vi "Actor Core.vi"(8 "error in":errorcluster, 11 "Apply Language Wizard in":refnum<class "Apply Language Wizard.lvclass">) -> (0 "error out":errorcluster, 3 "Actor out":refnum<class "Actor.lvclass">)   [LabVIEW 2013, in "SET Project Editor.lvlib" / "Apply Language Wizard.lvclass"]
doc: "(<B>Filename</B>: Actor Framework.lvlib:Actor.lvclass:Actor Core.vi)\n\nReceives messages to the actor, reacts to them, and initiates any error handling that may shut the actor down.\n\nDescendant classes may override this VI to append parallel tasks for the actor to complete while it handles messages. Overrides use the Call Parent Method node."
uses:
  Apply Language Wizard.lvclass
  <vilib>/ActorFramework/Actor/Actor.lvclass
  <vilib>/ActorFramework/Actor/Actor.lvclass/Actor.ctl
  <vilib>/ActorFramework/Message Enqueuer/Message Enqueuer.lvclass/Message Enqueuer.ctl
  Apply Language Wizard.lvclass/Apply Language Wizard.ctl
  lib/printf/messages/General/LV_Printf Msg.lvclass/LV_Printf Msg.ctl
  UI Wizard/UI Wizard.lvclass
  lib/printf/messages/General/Read Message.vi
  <vilib>/ActorFramework/Message Enqueuer/Init from Existing Queue.vi
  <vilib>/ActorFramework/Message Enqueuer/Enqueue.vi
  <vilib>/ActorFramework/Message Priority Queue/Priority Enqueue.vi
  <vilib>/ActorFramework/Message Enqueuer/Message Enqueuer.lvclass
  <vilib>/ActorFramework/Stop Msg/Stop Msg.lvclass
  Apply Language Wizard Messages/Apply Language to Project Msg/Apply Language to Project Msg.lvclass
  lib/printf/Core/LV_Printf Core.lvclass
  lib/printf/messages/General/LV_Printf Msg.lvclass
panel:
  in  "Tab Control":enum32{"Page 1", "Page 2"}(tab)
  in  "Next1":bool
  out "Project Name":string
  in  "Cancel1":bool
  in  "Target Language":string(combo)="en" caption="Default Language"
  in  "VI Selector":i32(listbox)
  in  "RTM Selector":i32(listbox)
  out "Status":string
  in  "Finish":bool
  in  "Cancel2":bool
  # "Apply Language Wizard"
  # "Select VIs"
  # "Select Run-Time Menus"
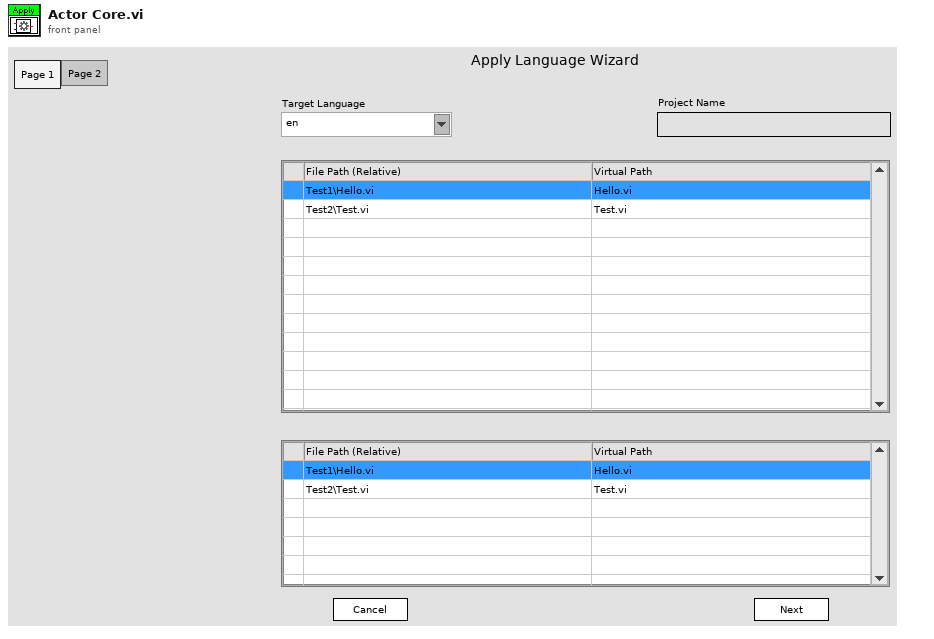
[diagram p1: front panel]
types:
  T1 = typedef "LVPoint32TypeDef.ctl" = cluster{"Horizontal":i32, "Vertical":i32}
  T2 = typedef "LVRowAndColumnTypeDef.ctl" = cluster{"Row":i32, "Column":i32}
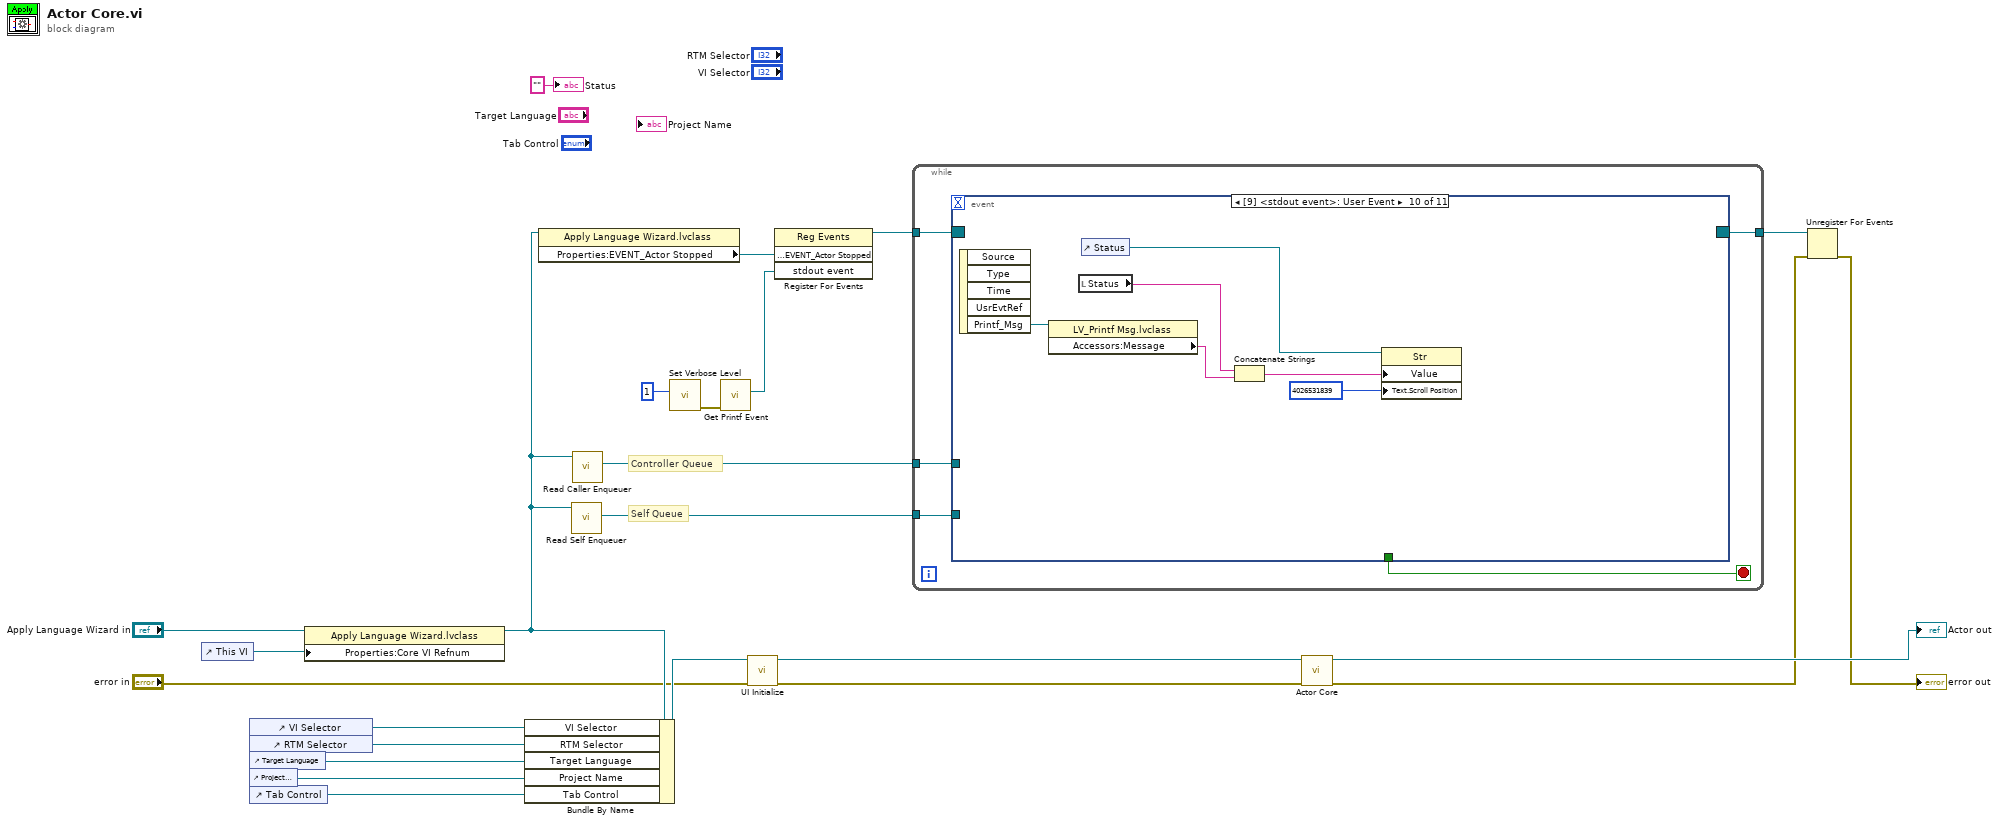
[diagram p0: block diagram]
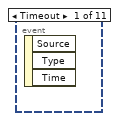
[diagram p2: hidden frame]
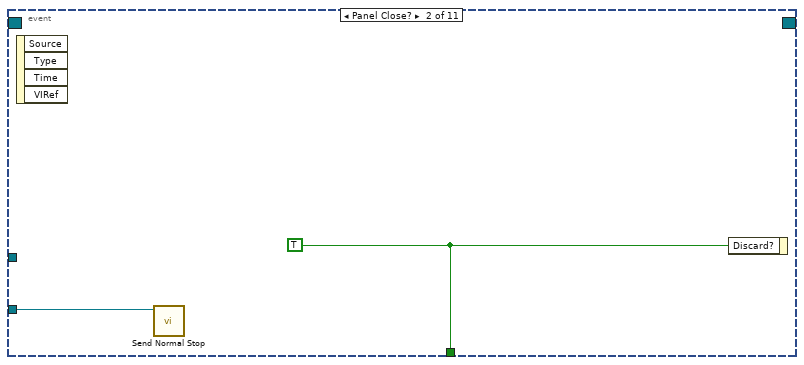
[diagram p3: hidden frame]
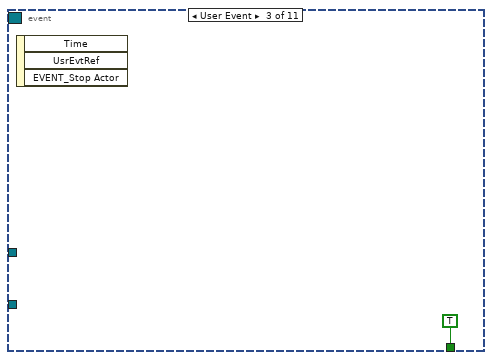
[diagram p4: hidden frame]
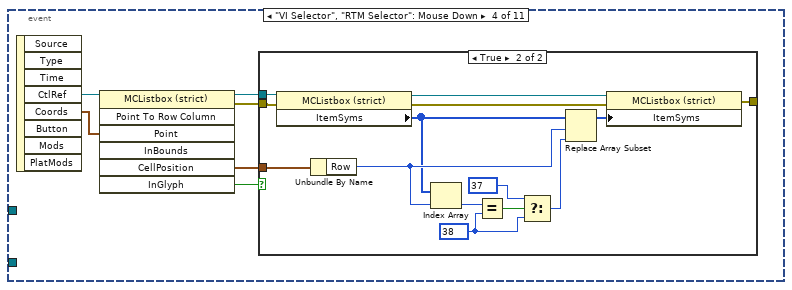
[diagram p5: hidden frame]
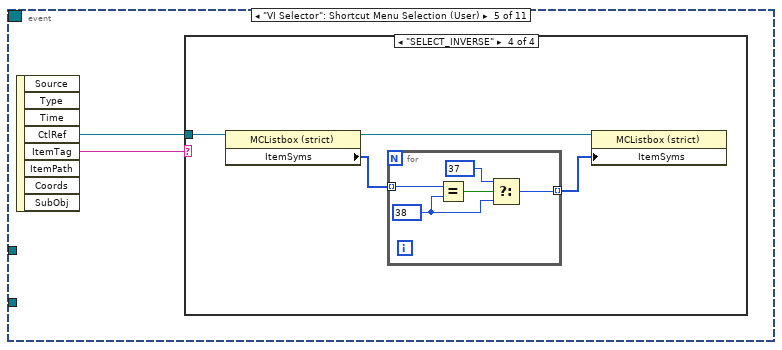
[diagram p7: hidden frame]
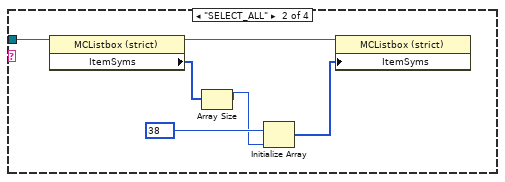
[diagram p9: hidden frame]
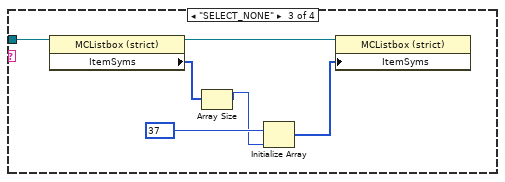
[diagram p10: hidden frame]
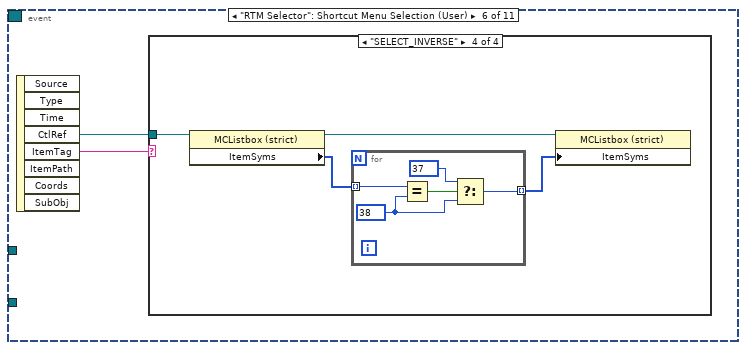
[diagram p11: hidden frame]
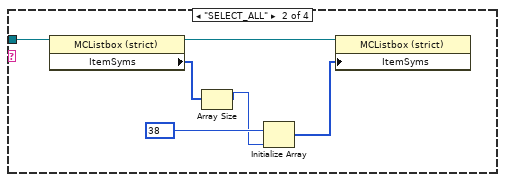
[diagram p13: hidden frame]
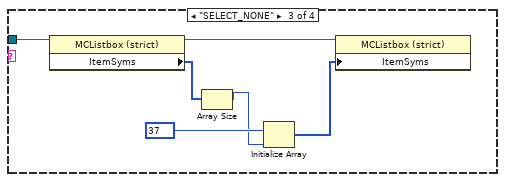
[diagram p14: hidden frame]
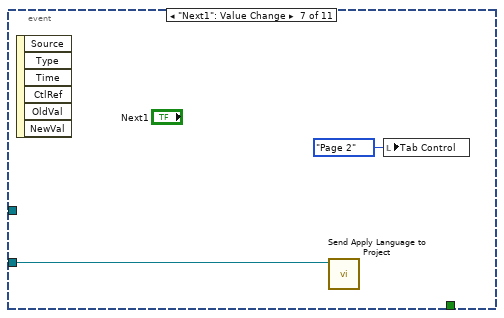
[diagram p15: hidden frame]
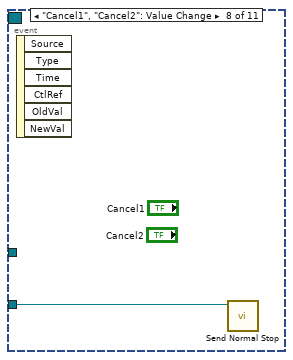
[diagram p16: hidden frame]
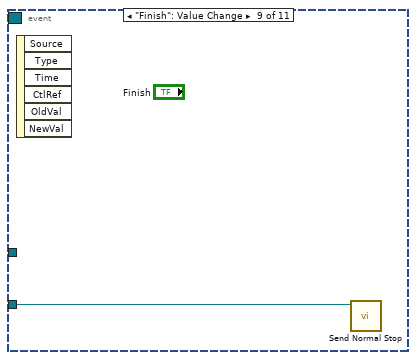
[diagram p17: hidden frame]
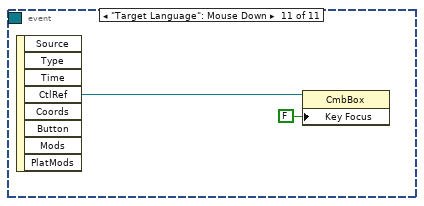
[diagram p18: hidden frame]
diagram:
  # "Controller Queue"
  # "Self Queue"
  n1 = control-ref of="This VI"() -> (w18:refnum<vi>)
  n2 = control-ref of="VI Selector"() -> (w3:refnum<vi>)
  n3 = control-ref of="RTM Selector"() -> (w4:refnum<vi>)
  n4 = control-ref of="Target Language"() -> (w5:refnum<vi>)
  n5 = control-ref of="Project Name"() -> (w2:refnum<vi>)
  n6 = control-ref of="Tab Control"() -> (w6:refnum<vi>)
  n7 = property class="Apply Language Wizard.lvclass"(reference="Apply Language Wizard in", "Properties:Core VI Refnum"=w18) -> (reference out=w9:refnum<class "Apply Language Wizard.lvclass">)  [unwired: 1 in, 1 out]
  n8 = Bundle By Name(cluster=w9, "VI Selector"=w3, "RTM Selector"=w4, "Target Language"=w5, "Project Name"=w2, "Tab Control"=w6) -> (w8:refnum<class "Apply Language Wizard.lvclass">)
  n9 = property class="Apply Language Wizard.lvclass"(reference=w9) -> ("Properties:EVENT_Actor Stopped"=w23:refnum<user-event>)  [unwired: 1 in, 2 out]
  n10 = call <vilib>:"Read Self Enqueuer.vi"("Actor"=w9) -> ("Self Enqueuer"=w14:refnum<class "Message Enqueuer.lvclass">)  [unwired: 10 in]
  n11 = call <vilib>:"Read Caller Enqueuer.vi"("Actor"=w9) -> ("Caller Enqueuer"=w15:refnum<class "Message Enqueuer.lvclass">)  [unwired: 10 in]
  n12 = call "Set Verbose Level.vi"("Verbose Level"=1) -> ("error out"=w21:errorcluster)  [unwired: 10 in]
  n13 = call "Get Printf Event.vi"("error in (no error)"=w21) -> ("stdout event"=w20:refnum<user-event>)  [unwired: 8 in, 2 out]
  n14 = call-dynamic "UI Initialize.vi"("error in (no error)"="error in", "Apply Language Wizard in"=w8) -> ("error out"=w10:errorcluster, "Apply Language Wizard out"=w11:refnum<class "Apply Language Wizard.lvclass">)  [unwired: 8 in]
  n15 = register-events(w23, w20) -> (reference out=w16:refnum<event-registration>)  [unwired: 2 in, 1 out]
  n16 = while {
    tunnel: w16 -> [w28]
    tunnel: [w27] -> w17
    tunnel: w14 -> [w26]
    tunnel: w15 -> [w25]
    stop <- w29 stop-if-true
    n17 = event shown="[9] <stdout event>: User Event" {
      selector: w28 -> [_ _ _ _ _ _ _ _ _ _ _]
      dyn-events: [_ _ _ _ _ _ _ _ _ _ _] -> w27
      timeout: _ -> [_ _ _ _ _ _ _ _ _ _ _]
      tunnel: [_ w31 TRUE ("Discard?") _ _ _ _ _ _ _ _] -> w29
      tunnel: w26 -> [_ w30 _ _ _ _ w101 w102 w103 _ _]
      tunnel: w25 -> [_ _ _ _ _ _ _ _ _ _ _]
      event Timeout {
        n18 = event-data() -> ()  [unwired: 1 in, 3 out]
      }
      event Panel Close? {
        w31 = TRUE ("Discard?")
        n19 = event-data() -> ()  [unwired: 1 in, 4 out]
        n20 = call <vilib>:"Send Normal Stop.vi"("Message Enqueuer"=w30) -> ()  [unwired: 10 in, 1 out]
        n21 = event-data("Discard?"=w31) -> ()  [unwired: 1 in, 1 out]
      }
      event User Event {
        n22 = event-data() -> ()  [unwired: 1 in, 3 out]
      }
      event "VI Selector", "RTM Selector": Mouse Down {
        n23 = event-data() -> ("CtlRef"=w34:refnum<vi>, "Coords"=w33:T1)  [unwired: 1 in, 6 out]
        n24 = invoke class="MCListbox (strict)" method="Point To Row Column"(reference=w34, "Point"=w33) -> (reference out=w36:refnum<vi>, error out=w37:errorcluster, "CellPosition"=w38:T2, "InGlyph"=w35:bool)  [unwired: 5 in, 3 out]
        n25 = case shown="True" w35 {
          tunnel: w38 -> [_ w53]
          tunnel: w37 -> [w39 w52]
          tunnel: [w39 w49] -> _
          tunnel: w36 -> [_ w48]
          frame False {
          }
          frame True {
            w44 = 38
            n26 = property on="Property Node" class="MCListbox (strict)"(reference=w48, error in=w52) -> (reference out=w47:refnum<vi>, error out=w51:errorcluster, "ItemSyms"=w41:i32[])
            n27 = Unbundle By Name(w53) -> ("Row"=w42:i32)
            n28 = Index Array(array=w41, index=w42) -> (element=w46:i32)
            n29 = Equal?(x=w46, y=w44) -> (x = y?=w45:bool)
            n30 = Select(t=37, s=w45, f=w44) -> (s? t:f=w43:i32)
            n31 = Replace Array Subset(array=w41, new element=w43, index=w42) -> (w50:i32[])
            n32 = property on="Property Node" class="MCListbox (strict)"(reference=w47, error in=w51, "ItemSyms"=w50) -> (error out=w49:errorcluster)  [unwired: 1 out]
          }
        }
      }
      event "VI Selector": Shortcut Menu Selection (User) {
        n33 = event-data() -> ("CtlRef"=w55:refnum<vi>, "ItemTag"=w54:string)  [unwired: 1 in, 6 out]
        n34 = case shown="\"SELECT_INVERSE\"" w54 {
          tunnel: w55 -> [_ w61 w67 w71]
          frame "False", Default {
          }
          frame "SELECT_ALL" {
            n35 = property class="MCListbox (strict)"(reference=w61) -> (reference out=w56:refnum<vi>, "ItemSyms"=w60:i32[])  [unwired: 1 in, 1 out]
            n36 = Array Size(array=w60) -> (size(s)=w58:i32)
            n37 = Initialize Array(38, w58) -> (w57:i32[])
            n38 = property class="MCListbox (strict)"(reference=w56, "ItemSyms"=w57) -> ()  [unwired: 1 in, 2 out]
          }
          frame "SELECT_NONE" {
            n39 = property class="MCListbox (strict)"(reference=w67) -> (reference out=w62:refnum<vi>, "ItemSyms"=w66:i32[])  [unwired: 1 in, 1 out]
            n40 = Array Size(array=w66) -> (size(s)=w64:i32)
            n41 = Initialize Array(37, w64) -> (w63:i32[])
            n42 = property class="MCListbox (strict)"(reference=w62, "ItemSyms"=w63) -> ()  [unwired: 1 in, 2 out]
          }
          frame "SELECT_INVERSE" {
            n43 = property class="MCListbox (strict)"(reference=w71) -> (reference out=w70:refnum<vi>, "ItemSyms"=w69:i32[])  [unwired: 1 in, 1 out]
            n44 = for {
              tunnel: w69 -> [w76] mode=indexing
              tunnel: [w72] -> w68 mode=indexing
              w73 = 38
              n45 = Equal?(x=w76, y=w73) -> (x = y?=w75:bool)
              n46 = Select(t=37, s=w75, f=w73) -> (s? t:f=w72:i32)
            }
            n47 = property class="MCListbox (strict)"(reference=w70, "ItemSyms"=w68) -> ()  [unwired: 1 in, 2 out]
          }
        }
      }
      event "RTM Selector": Shortcut Menu Selection (User) {
        n48 = event-data() -> ("CtlRef"=w78:refnum<vi>, "ItemTag"=w77:string)  [unwired: 1 in, 6 out]
        n49 = case shown="\"SELECT_INVERSE\"" w77 {
          tunnel: w78 -> [_ w84 w90 w94]
          frame "False", Default {
          }
          frame "SELECT_ALL" {
            n50 = property class="MCListbox (strict)"(reference=w84) -> (reference out=w79:refnum<vi>, "ItemSyms"=w83:i32[])  [unwired: 1 in, 1 out]
            n51 = Array Size(array=w83) -> (size(s)=w81:i32)
            n52 = Initialize Array(38, w81) -> (w80:i32[])
            n53 = property class="MCListbox (strict)"(reference=w79, "ItemSyms"=w80) -> ()  [unwired: 1 in, 2 out]
          }
          frame "SELECT_NONE" {
            n54 = property class="MCListbox (strict)"(reference=w90) -> (reference out=w85:refnum<vi>, "ItemSyms"=w89:i32[])  [unwired: 1 in, 1 out]
            n55 = Array Size(array=w89) -> (size(s)=w87:i32)
            n56 = Initialize Array(37, w87) -> (w86:i32[])
            n57 = property class="MCListbox (strict)"(reference=w85, "ItemSyms"=w86) -> ()  [unwired: 1 in, 2 out]
          }
          frame "SELECT_INVERSE" {
            n58 = property class="MCListbox (strict)"(reference=w94) -> (reference out=w93:refnum<vi>, "ItemSyms"=w92:i32[])  [unwired: 1 in, 1 out]
            n59 = for {
              tunnel: w92 -> [w99] mode=indexing
              tunnel: [w95] -> w91 mode=indexing
              w96 = 38
              n60 = Equal?(x=w99, y=w96) -> (x = y?=w98:bool)
              n61 = Select(t=37, s=w98, f=w96) -> (s? t:f=w95:i32)
            }
            n62 = property class="MCListbox (strict)"(reference=w93, "ItemSyms"=w91) -> ()  [unwired: 1 in, 2 out]
          }
        }
      }
      event "Next1": Value Change {
        n63 = event-data() -> ()  [unwired: 1 in, 6 out]
        n64 = call "Send Apply Language to Project.vi"("Message Enqueuer"=w101) -> ()  [unwired: 9 in, 2 out]
        n65 = local write "Tab Control"(enum32{"Page 1", "Page 2"}."Page 2" ("Tab Control")) -> ()
      }
      event "Cancel1", "Cancel2": Value Change {
        n66 = event-data() -> ()  [unwired: 1 in, 6 out]
        n67 = call <vilib>:"Send Normal Stop.vi"("Message Enqueuer"=w102) -> ()  [unwired: 10 in, 1 out]
      }
      event "Finish": Value Change {
        n68 = event-data() -> ()  [unwired: 1 in, 6 out]
        n69 = call <vilib>:"Send Normal Stop.vi"("Message Enqueuer"=w103) -> ()  [unwired: 10 in, 1 out]
      }
      event User Event {
        n70 = event-data() -> ("Printf_Msg"=w107:refnum<class "LV_Printf Msg.lvclass">)  [unwired: 1 in, 4 out]
        n71 = property class="LV_Printf Msg.lvclass"(reference=w107) -> ("Accessors:Message"=w105:string)  [unwired: 1 in, 2 out]
        n72 = local read "Status"() -> (w106:string)
        n73 = control-ref of="Status"() -> (w109:refnum<vi>)
        n74 = Concatenate Strings(w106, w105) -> (w104:string)
        n75 = property class="Str"(reference=w109, "Value"=w104, "Text.Scroll Position"=u32 4026531839) -> ()  [unwired: 1 in, 2 out]
      }
      event "Target Language": Mouse Down {
        n76 = event-data() -> ("CtlRef"=w111:refnum<vi>)  [unwired: 1 in, 7 out]
        n77 = property class="CmbBox"(reference=w111, "Key Focus"=FALSE) -> ()  [unwired: 1 in, 2 out]
      }
    }
  }
  n78 = call-parent "Actor Core.vi"("error in"=w10, "Actor in"=w11) -> ("error out"=w13:errorcluster, "Actor out"=→"Actor out":refnum<class "Actor.lvclass">)  [unwired: 8 in]
  n79 = Unregister For Events(event registration refnum=w17, error in=w13) -> (error out=→"error out":errorcluster)
  "Status" <- "" ("Status")
